vi "Double Sided Spectrum.vi"(8 "Error In":errorcluster, 11 "Signals In":waveform(dbl)[](array[waveform])) -> (0 "Error Out":errorcluster, 3 "Double Sided Spectra":cluster{"f0":dbl, "df":dbl, "magnitude":dbl[]}[](array[cluster]))   [LabVIEW 2020]
uses:
  <vilib>/Analysis/2dsp.llb/Real FFT.vi
  <vilib>/Analysis/NI_AALPro.lvlib
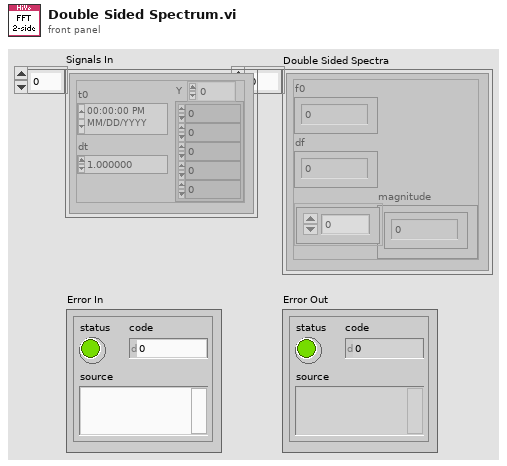
[diagram p1: front panel]
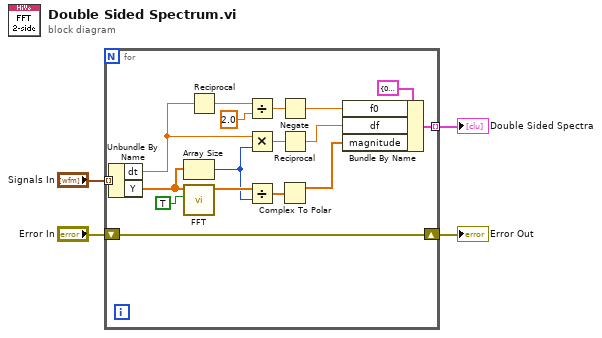
[diagram p0: block diagram]
diagram:
  n1 = for {
    tunnel: [w15] -> w4 mode=indexing
    tunnel: "Signals In" -> [w10] mode=indexing
    shift-right: [w5] -> w1
    shift-left: "Error In" -> [w5]
    n2 = Unbundle By Name(w10) -> ("dt"=w18:dbl, "Y"=w11:dbl[])
    n3 = Array Size(array=w11) -> (size(s)=w7:i32)
    n4 = call-poly <vilib>:"FFT.vi"("shift?"=TRUE, "X"=w11) -> ("FFT {X}"=w9:cdb[])  [unwired: 8 in, 1 out]
    n5 = Reciprocal(x=w18) -> (1/x=w19:dbl)
    n6 = Divide(x=w19, y=2.0) -> (x/y=w21:dbl)
    n7 = Multiply(x=w18, y=w7) -> (x*y=w12:dbl)
    n8 = Divide(x=w9, y=w7) -> (x/y=w8:cdb[])
    n9 = Negate(x=w21) -> (-x=w6:dbl)
    n10 = Reciprocal(x=w12) -> (1/x=w13:dbl)
    n11 = Complex To Polar(r * e^(i*theta)=w8) -> (r=w14:dbl[])  [unwired: 1 out]
    n12 = Bundle By Name(cluster=cluster{"f0":dbl, "df":dbl, "magnitude":dbl[]} {"f0"=0.0, "df"=0.0, "magnitude"=[]} ("input cluster"), "f0"=w6, "df"=w13, "magnitude"=w14) -> (w15:cluster{"f0":dbl, "df":dbl, "magnitude":dbl[]})
  }
  "Double Sided Spectra" <- w4
  "Error Out" <- w1
